vi "DoesNothing.vi"(8 "error in (no error)":errorcluster) -> (0 "error out":errorcluster)   [LabVIEW 2020]
uses:
  Auxilary/AuxGlobals.vi
  DriveSystem/DriveGlobals.vi
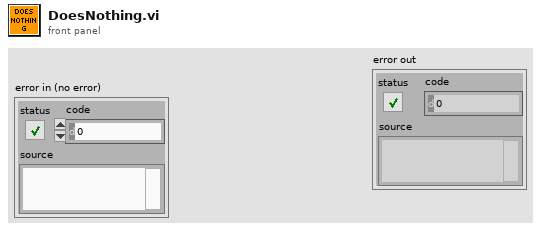
[diagram p1: front panel]
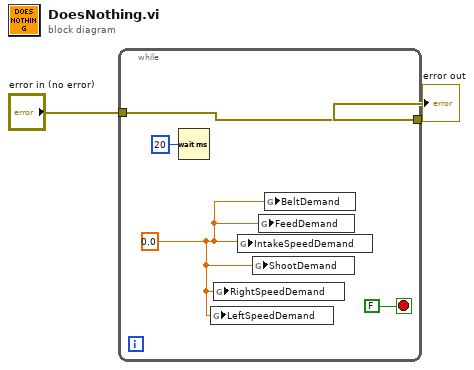
[diagram p0: block diagram]
diagram:
  n1 = while {
    tunnel: [w5] -> w2
    tunnel: "error in (no error)" -> [w5]
    stop <- FALSE stop-if-true
    w3 = 0.0
    n2 = Wait (ms)(milliseconds to wait=u32 20) -> ()  [unwired: 1 out]
    n3 = global write "DriveGlobals.vi" "LeftSpeedDemand"(w3) -> ()
    n4 = global write "DriveGlobals.vi" "RightSpeedDemand"(w3) -> ()
    n5 = global write "AuxGlobals.vi" "IntakeSpeedDemand"(w3) -> ()
    n6 = global write "AuxGlobals.vi" "ShootDemand"(w3) -> ()
    n7 = global write "AuxGlobals.vi" "FeedDemand"(w3) -> ()
    n8 = global write "AuxGlobals.vi" "BeltDemand"(w3) -> ()
  }
  "error out" <- w2
